vi "Mock Generation Demo.vi"() -> ()   [LabVIEW 2020]
uses:
  source/Scripting/Mock Class Generator/Mock Class Generator.lvclass
panel:
  out "error out":errorcluster
  in  "Destination Class Path":path
  in  "Source Class":path
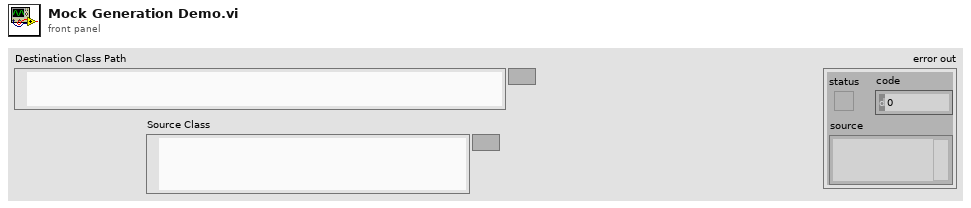
[diagram p1: front panel]
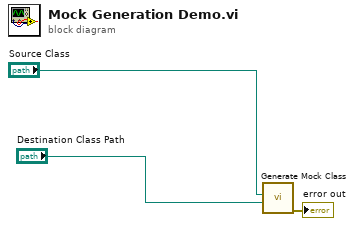
[diagram p0: block diagram]
diagram:
  n1 = call "Generate Mock Class.vi"("Destination Class Path"="Destination Class Path", "Source Class Path"="Source Class") -> ("error out"=→"error out":errorcluster)  [unwired: 9 in]
